vi "Sort Dot Positions ver2.vi"(1 "Present Position (input)":T1 {"Point3" format="%.2f"; "Point2" format="%.2f"; "Point1" format="%.2f"}, 2 "Previous Position":T1 {"Point3" format="%.2f"; "Point2" format="%.2f"; "Point1" format="%.2f"}) -> (0 "Present Position (output)":T1 {"Point3" format="%.2f"; "Point2" format="%.2f"; "Point1" format="%.2f"})   [LabVIEW 2013, in "3 dot tracker.lvlib"]
uses:
  3 dot tracker.lvlib
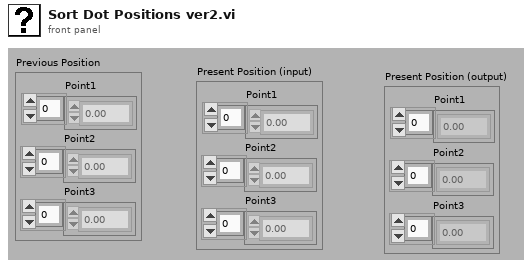
[diagram p1: front panel]
types:
  T1 = cluster{"Point1":dbl[], "Point2":dbl[], "Point3":dbl[]}
  T2 = cluster{"Point3":dbl[], "Point1":dbl[], "Point2":dbl[]}
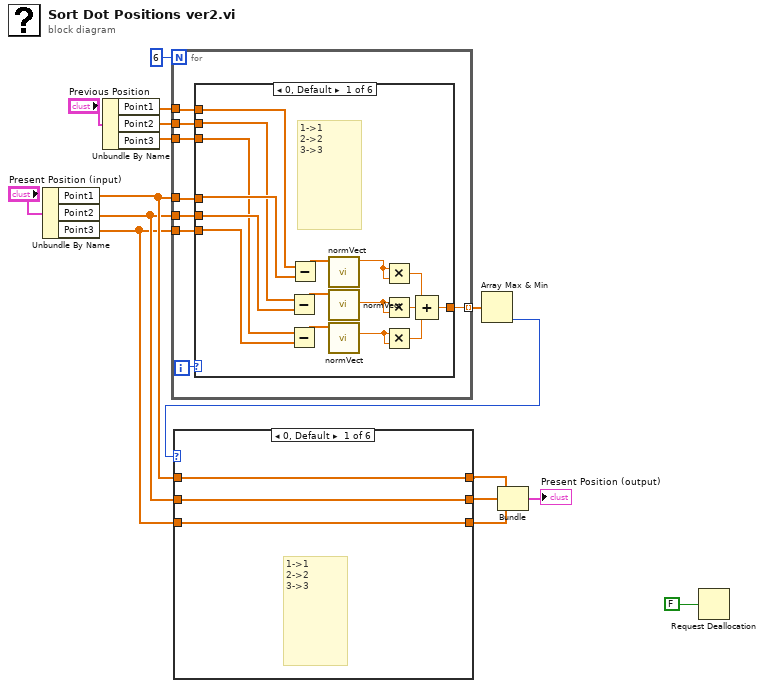
[diagram p0: block diagram]
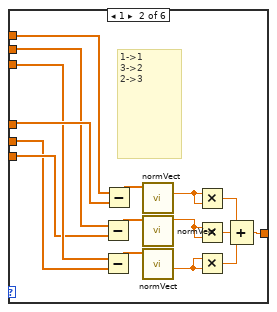
[diagram p7: hidden frame]
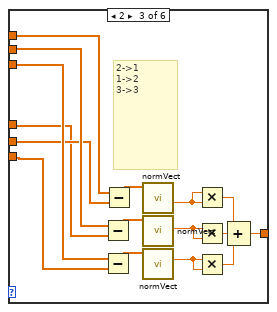
[diagram p8: hidden frame]
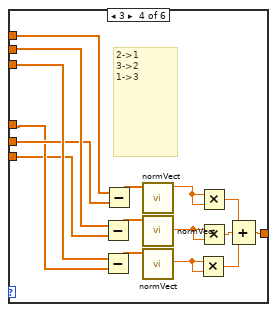
[diagram p9: hidden frame]
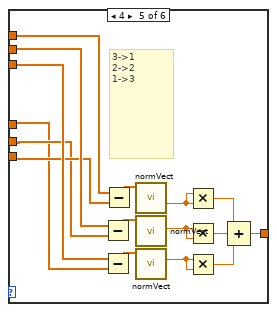
[diagram p10: hidden frame]
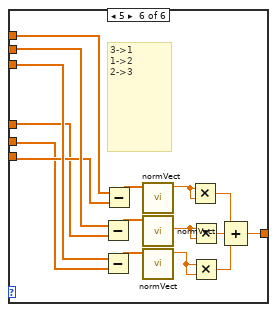
[diagram p11: hidden frame]
diagram:
  n1 = Unbundle By Name("Present Position (input)") -> ("Point1"=w8:dbl[], "Point2"=w7:dbl[], "Point3"=w6:dbl[])
  n2 = Unbundle By Name("Previous Position") -> ("Point1"=w13:dbl[], "Point2"=w12:dbl[], "Point3"=w11:dbl[])
  n3 = for {
    N: 6 -> [_]
    tunnel: w13 -> [w23]
    tunnel: w12 -> [w21]
    tunnel: w11 -> [w20]
    tunnel: w8 -> [w24]
    tunnel: w7 -> [w19]
    tunnel: w6 -> [w18]
    tunnel: [w17] -> w2 mode=indexing
    i -> [w22]
    n4 = case shown="0, Default" w22 {
      tunnel: w24 -> [w40 w56 w63 w80 w95 w112]
      tunnel: w23 -> [w39 w55 w72 w88 w104 w120]
      tunnel: w21 -> [w38 w54 w71 w87 w103 w119]
      tunnel: w20 -> [w36 w53 w70 w86 w102 w118]
      tunnel: w19 -> [w37 w47 w64 w81 w96 w111]
      tunnel: w18 -> [w35 w48 w65 w79 w97 w113]
      tunnel: [w31 w49 w66 w82 w98 w114] -> w17
      frame 0, Default {
        # "1->1\n2->2\n3->3"
        n5 = Subtract(x=w38, y=w37) -> (x-y=w33:dbl[])
        n6 = Subtract(x=w36, y=w35) -> (x-y=w32:dbl[])
        n7 = Subtract(x=w39, y=w40) -> (x-y=w34:dbl[])
        n8 = call "normVect.vi"("Array"=w34) -> ("norm"=w27:dbl)  [unwired: 10 in]
        n9 = call "normVect.vi"("Array"=w33) -> ("norm"=w26:dbl)  [unwired: 10 in]
        n10 = call "normVect.vi"("Array"=w32) -> ("norm"=w25:dbl)  [unwired: 10 in]
        n11 = Multiply(x=w27, y=w27) -> (x*y=w30:dbl)
        n12 = Multiply(x=w26, y=w26) -> (x*y=w29:dbl)
        n13 = Multiply(x=w25, y=w25) -> (x*y=w28:dbl)
        n14 = Compound Arithmetic op=ADD(w30, w29, w28) -> (w31:dbl)
      }
      frame 1 {
        # "1->1\n3->2\n2->3"
        n15 = Subtract(x=w54, y=w48) -> (x-y=w51:dbl[])
        n16 = Subtract(x=w53, y=w47) -> (x-y=w50:dbl[])
        n17 = Subtract(x=w55, y=w56) -> (x-y=w52:dbl[])
        n18 = call "normVect.vi"("Array"=w52) -> ("norm"=w43:dbl)  [unwired: 10 in]
        n19 = call "normVect.vi"("Array"=w51) -> ("norm"=w42:dbl)  [unwired: 10 in]
        n20 = call "normVect.vi"("Array"=w50) -> ("norm"=w41:dbl)  [unwired: 10 in]
        n21 = Multiply(x=w43, y=w43) -> (x*y=w46:dbl)
        n22 = Multiply(x=w42, y=w42) -> (x*y=w45:dbl)
        n23 = Multiply(x=w41, y=w41) -> (x*y=w44:dbl)
        n24 = Compound Arithmetic op=ADD(w46, w45, w44) -> (w49:dbl)
      }
      frame 2 {
        # "2->1\n1->2\n3->3"
        n25 = Subtract(x=w71, y=w63) -> (x-y=w68:dbl[])
        n26 = Subtract(x=w70, y=w65) -> (x-y=w67:dbl[])
        n27 = Subtract(x=w72, y=w64) -> (x-y=w69:dbl[])
        n28 = call "normVect.vi"("Array"=w69) -> ("norm"=w59:dbl)  [unwired: 10 in]
        n29 = call "normVect.vi"("Array"=w68) -> ("norm"=w58:dbl)  [unwired: 10 in]
        n30 = call "normVect.vi"("Array"=w67) -> ("norm"=w57:dbl)  [unwired: 10 in]
        n31 = Multiply(x=w59, y=w59) -> (x*y=w62:dbl)
        n32 = Multiply(x=w58, y=w58) -> (x*y=w61:dbl)
        n33 = Multiply(x=w57, y=w57) -> (x*y=w60:dbl)
        n34 = Compound Arithmetic op=ADD(w62, w61, w60) -> (w66:dbl)
      }
      frame 3 {
        # "2->1\n3->2\n1->3"
        n35 = Subtract(x=w87, y=w79) -> (x-y=w84:dbl[])
        n36 = Subtract(x=w86, y=w80) -> (x-y=w83:dbl[])
        n37 = Subtract(x=w88, y=w81) -> (x-y=w85:dbl[])
        n38 = call "normVect.vi"("Array"=w85) -> ("norm"=w75:dbl)  [unwired: 10 in]
        n39 = call "normVect.vi"("Array"=w84) -> ("norm"=w74:dbl)  [unwired: 10 in]
        n40 = call "normVect.vi"("Array"=w83) -> ("norm"=w73:dbl)  [unwired: 10 in]
        n41 = Multiply(x=w73, y=w73) -> (x*y=w76:dbl)
        n42 = Multiply(x=w75, y=w75) -> (x*y=w78:dbl)
        n43 = Multiply(x=w74, y=w74) -> (x*y=w77:dbl)
        n44 = Compound Arithmetic op=ADD(w78, w77, w76) -> (w82:dbl)
      }
      frame 4 {
        # "3->1\n2->2\n1->3"
        n45 = Subtract(x=w103, y=w96) -> (x-y=w100:dbl[])
        n46 = Subtract(x=w102, y=w95) -> (x-y=w99:dbl[])
        n47 = Subtract(x=w104, y=w97) -> (x-y=w101:dbl[])
        n48 = call "normVect.vi"("Array"=w101) -> ("norm"=w93:dbl)  [unwired: 10 in]
        n49 = call "normVect.vi"("Array"=w100) -> ("norm"=w91:dbl)  [unwired: 10 in]
        n50 = call "normVect.vi"("Array"=w99) -> ("norm"=w89:dbl)  [unwired: 10 in]
        n51 = Multiply(x=w93, y=w93) -> (x*y=w94:dbl)
        n52 = Multiply(x=w91, y=w91) -> (x*y=w92:dbl)
        n53 = Multiply(x=w89, y=w89) -> (x*y=w90:dbl)
        n54 = Compound Arithmetic op=ADD(w94, w92, w90) -> (w98:dbl)
      }
      frame 5 {
        # "3->1\n1->2\n2->3"
        n55 = Subtract(x=w119, y=w112) -> (x-y=w116:dbl[])
        n56 = Subtract(x=w118, y=w111) -> (x-y=w115:dbl[])
        n57 = Subtract(x=w120, y=w113) -> (x-y=w117:dbl[])
        n58 = call "normVect.vi"("Array"=w117) -> ("norm"=w109:dbl)  [unwired: 10 in]
        n59 = call "normVect.vi"("Array"=w116) -> ("norm"=w107:dbl)  [unwired: 10 in]
        n60 = call "normVect.vi"("Array"=w115) -> ("norm"=w105:dbl)  [unwired: 10 in]
        n61 = Multiply(x=w109, y=w109) -> (x*y=w110:dbl)
        n62 = Multiply(x=w107, y=w107) -> (x*y=w108:dbl)
        n63 = Multiply(x=w105, y=w105) -> (x*y=w106:dbl)
        n64 = Compound Arithmetic op=ADD(w110, w108, w106) -> (w114:dbl)
      }
    }
  }
  n65 = Array Max & Min(array=w2) -> (min index (indices)=w9:i32)  [unwired: 3 out]
  n66 = case shown="0, Default" w9 {
    tunnel: w8 -> [w123 w126 w127 w130 w133 w137]
    tunnel: w7 -> [w122 w124 w128 w132 w135 w136]
    tunnel: w6 -> [w121 w125 w129 w131 w134 w138]
    tunnel: [w123 w126 w128 w132 w134 w138] -> w5
    tunnel: [w122 w125 w127 w131 w135 w137] -> w4
    tunnel: [w121 w124 w129 w130 w133 w136] -> w3
    frame 0, Default {
      # "1->1\n2->2\n3->3"
    }
    frame 1 {
      # "1->1\n3->2\n2->3"
    }
    frame 2 {
      # "2->1\n1->2\n3->3"
    }
    frame 3 {
      # "2->1\n3->2\n1->3"
    }
    frame 4 {
      # "3->1\n2->2\n1->3"
    }
    frame 5 {
      # "3->1\n1->2\n2->3"
    }
  }
  n67 = Bundle("Point3"=w5, "Point1"=w4, "Point2"=w3) -> (→"Present Position (output)":T2)  [unwired: 1 in]
  n68 = Request Deallocation(FALSE ("flag")) -> ()
